vi "MPL.vi"(0 "System no.":i32=1 min=1 max=4 step=1, 2 "Affected axes":string[](array[string]), 3 "All axes?":bool, 5 "error in":errorcluster, 12 "Stop refnum":refnum<vi>) -> (14 "MPL successful?":bool[](array[boolean]), 19 "error out":errorcluster)   [LabVIEW 2020]
doc: "Moves specified axes to the positive limit switch, waits until this position is reached using #7 polling and indicates whether this was successful or not. VI will also stop if Stop refnum or Local stop is TRUE."
panel:
  in  "Local stop":bool
  # "Moves specified axes to the positive limit switch, waits until\nthis position is reached using #7 polling and indicates whether\nthis was successful or not. VI will also stop if Stop refnum or \nLocal stop is TRUE."
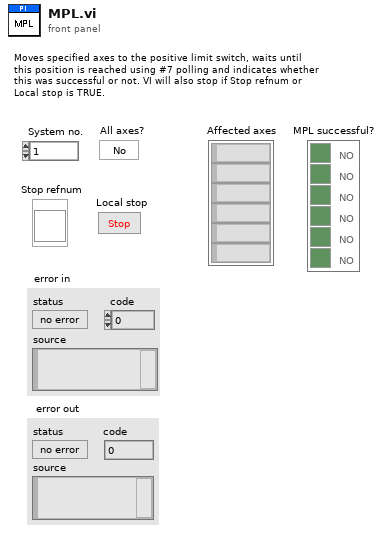
[diagram p1: front panel]
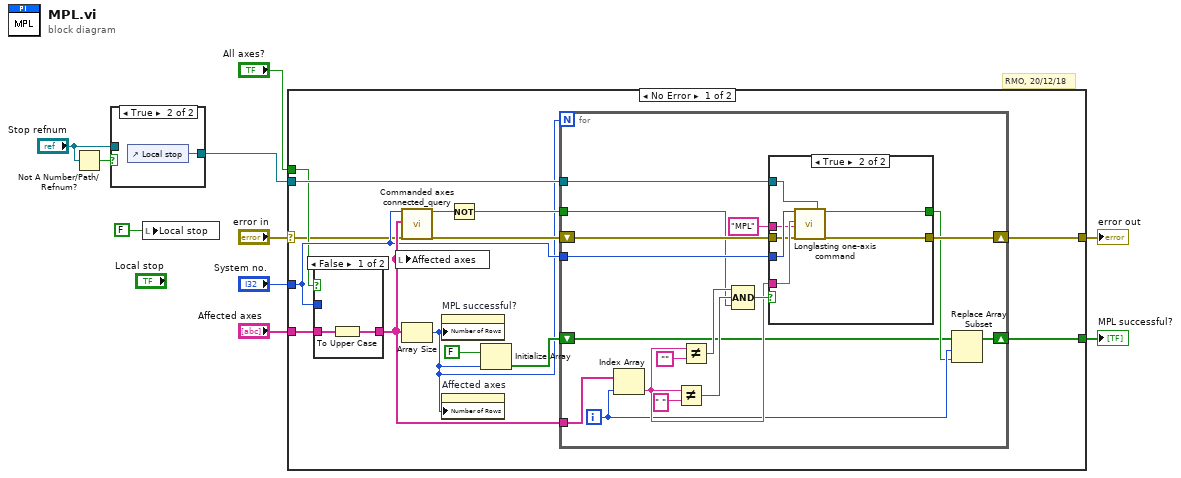
[diagram p0: block diagram]
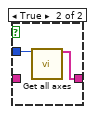
[diagram p3: hidden frame]
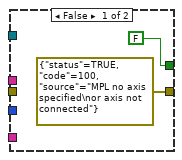
[diagram p4: hidden frame]
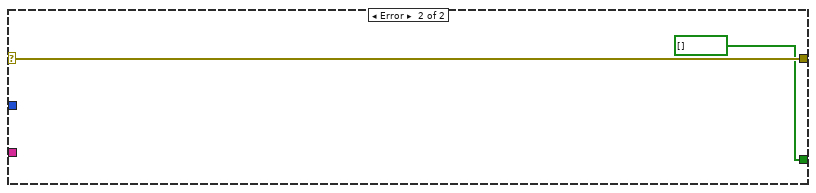
[diagram p5: hidden frame]
diagram:
  # "RMO, 20/12/18"
  n1 = Not A Number/Path/Refnum?(number/path/refnum="Stop refnum") -> (NaN/Path/Refnum?=w6:bool)
  n2 = case shown="True" w6 {
    tunnel: [w11 w12] -> w4
    tunnel: "Stop refnum" -> [w11 _]
    frame False {
    }
    frame True {
      n3 = control-ref of="Local stop"() -> (w12:refnum<vi>)
    }
  }
  n4 = local write "Local stop"(FALSE ("Local stop")) -> ()
  n5 = case shown="No Error" "error in" {
    selector: "error in" -> [w15 w58]
    tunnel: "All axes?" -> [w17 _]
    tunnel: "System no." -> [w18 _]
    tunnel: [w21 w58] -> w8
    tunnel: w4 -> [w20 _]
    tunnel: [w14 bool[] []] -> w2
    tunnel: "Affected axes" -> [w13 _]
    frame No Error {
      n6 = case shown="False" w17 {
        tunnel: [w28 w30] -> w19
        tunnel: w18 -> [_ w29]
        tunnel: w13 -> [w27 _]
        frame False {
          n7 = To Upper Case(1:w27) -> (0:w28:string[])
        }
        frame True {
          n8 = call "Get all axes.vi"("System no."=w29) -> ("Conn. Axes"=w30:string[])  [unwired: 18 out]
        }
      }
      n9 = local write "Affected axes"(w19) -> ()
      n10 = call "Commanded axes connected_query.vi"("System no."=w18, "Commanded axes"=w19, "error in"=w15) -> ("Controller error"=w23:bool, "error out"=w24:errorcluster)  [unwired: 15 out]
      n11 = Array Size(array=w19) -> (size(s)=w16:i32)
      n12 = property on="MPL successful?" class="Arr (strict)"("Number of Rows"=w16) -> ()  [unwired: 2 in, 2 out]
      n13 = property on="Affected axes" class="Arr (strict)"("Number of Rows"=w16) -> ()  [unwired: 2 in, 2 out]
      n14 = Not(x=w23) -> (.not. x?=w22:bool)
      n15 = Initialize Array(FALSE, w16) -> (w25:bool[])
      n16 = for {
        N: w16 -> [_]
        tunnel: w19 -> [w47]
        tunnel: w18 -> [w41]
        shift-right: [w39] -> w21
        shift-left: w24 -> [w38]
        shift-right: [w33] -> w14
        shift-left: w25 -> [w34]
        tunnel: w22 -> [w32]
        tunnel: w20 -> [w31]
        i -> [w36]
        n17 = Index Array(array=w47, index=w36) -> (element=w40:string)
        n18 = Not Equal?(x=w40, y=" ") -> (x != y?=w43:bool)
        n19 = Not Equal?(x=w40, y="") -> (x != y?=w44:bool)
        n20 = Compound Arithmetic op=AND(w44, w43, w32) -> (w42:bool)
        n21 = case shown="True" w42 {
          tunnel: w41 -> [_ w56]
          tunnel: w40 -> [_ w55]
          tunnel: [errorcluster {"status"=TRUE, "code"=100, "source"="MPL no axis specified\nor axis not connected"} ("error out") w54] -> w39
          tunnel: w38 -> [_ w53]
          tunnel: "MPL" -> [_ w52]
          tunnel: [FALSE w51] -> w35
          tunnel: w31 -> [_ w50]
          frame False {
          }
          frame True {
            n22 = call "Longlasting one-axis command.vi"("System no."=w56, "Axis to command"=w55, "Command"=w52, "error in"=w53, "Stop refnum"=w50) -> ("Answer"=w51:bool, "error out"=w54:errorcluster)  [unwired: 2 in, 11 out]
          }
        }
        n23 = Replace Array Subset(array=w34, new element=w35, index=w36) -> (w33:bool[])
      }
    }
    frame Error {
    }
  }
  "error out" <- w8
  "MPL successful?" <- w2
